vi "RPC Method package_service_method logic.vi"(8 "error in (no error)":errorcluster, 10 "gRPCid in":T1, 11 "OOP Server in":refnum<class "ServiceName.lvclass">) -> (0 "error out":errorcluster, 3 "OOP Server out":refnum<class "ServiceName.lvclass">)   [LabVIEW 2019, in "Service Template.lvlib" / "ServiceName.lvclass"]
uses:
  ServiceName.lvclass
  <vilib>/gRPC/LabVIEW gRPC Library/Server API/typeDefs/grpcId.ctl
  RPC Messages/package_templatemessage_Data.ctl
  Service Template.lvlib
  <vilib>/gRPC/LabVIEW gRPC Library/gprc-lvsupport-release.lvlib
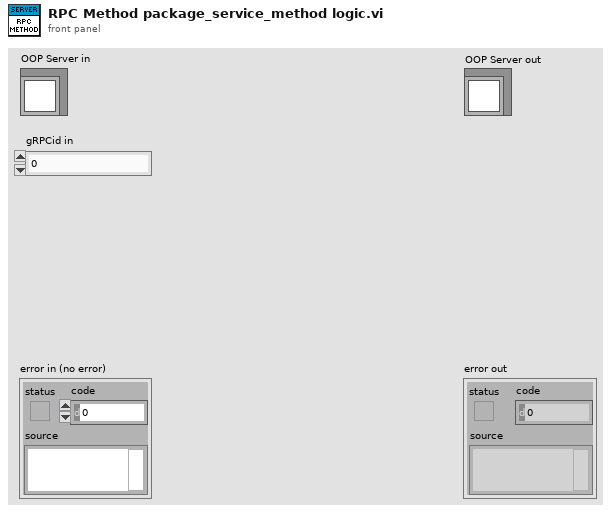
[diagram p1: front panel]
types:
  T1 = typedef "gprc-lvsupport-release.lvlib/grpcId.ctl" = u64
  T2 = typedef "Service Template.lvlib/package_templatemessage_Data.ctl" = cluster{"data":sgl}
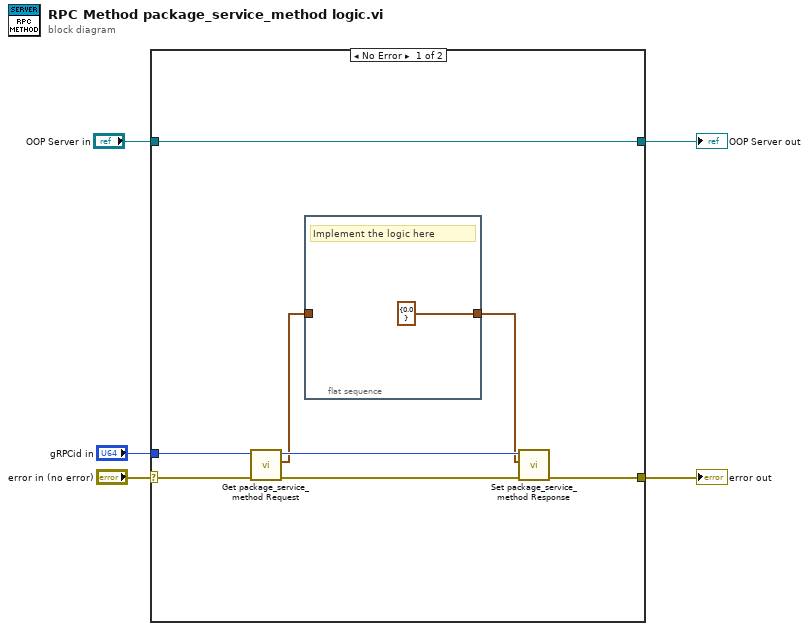
[diagram p0: block diagram]
diagram:
  n1 = case shown="No Error" "error in (no error)" {
    selector: "error in (no error)" -> [w12 w16]
    tunnel: [w10 w16] -> w4
    tunnel: "OOP Server in" -> [w13 w15]
    tunnel: [w13 w15] -> w2
    tunnel: "gRPCid in" -> [w8 _]
    frame No Error {
      n2 = call "Get package_service_method Request.vi"("error in (no error)"=w12, "gRPCid in"=w8) -> ("error out"=w11:errorcluster, "Message Data"=w7:T2, "gRPCid out"=w9:T1)  [unwired: 7 in]
      n3 = flat-sequence {
        tunnel: w7 -> [_]
        tunnel: [T2 {"data"=0.0} ("Message Data")] -> w6
        frame #0 {
          # "Implement the logic here"
        }
      }
      n4 = call "Set package_service_method Response.vi"("error in (no error)"=w11, "Message Data"=w6, "gRPCid in"=w9) -> ("error out"=w10:errorcluster)  [unwired: 8 in]
    }
    frame Error {
    }
  }
  "error out" <- w4
  "OOP Server out" <- w2
